vi "threshold-icator -scany.vi"(6 "first time":bool=TRUE, 7 "requested size":i32=1, 10 "gamma":dbl, 11 "omega":dbl) -> (0 "last peak":dbl, 1 "new peak":bool, 2 "gamma array":dbl[](array[numeric]), 3 "omega array":dbl[](array[numeric]))   [LabVIEW 2010]
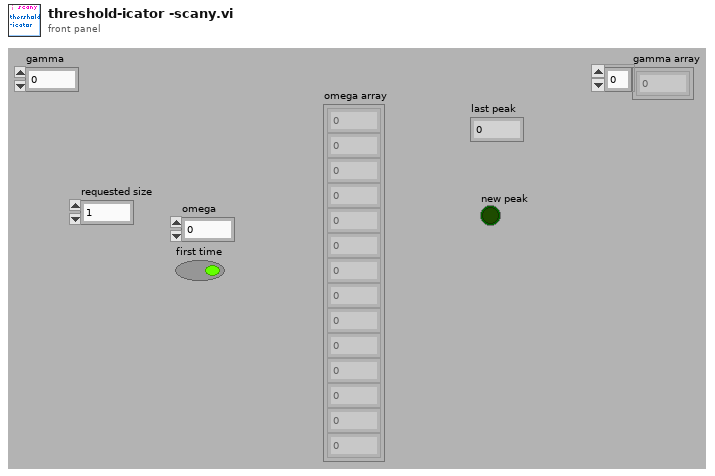
[diagram p1: front panel]
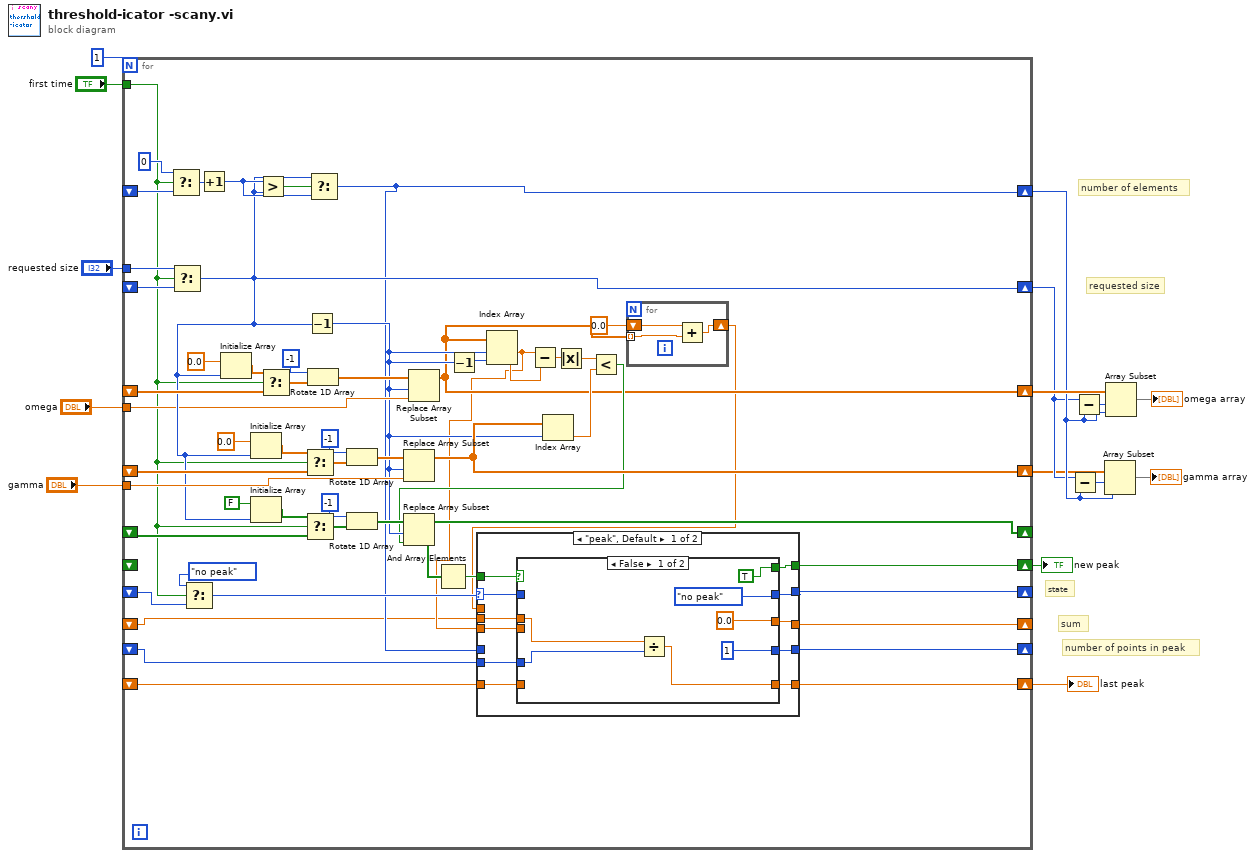
[diagram p0: block diagram]
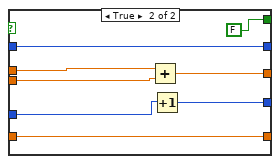
[diagram p2: hidden frame]
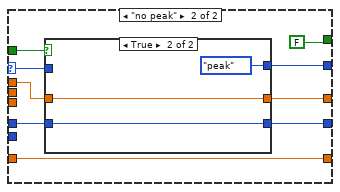
[diagram p3: hidden frame]
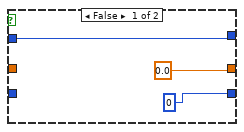
[diagram p4: hidden frame]
diagram:
  # "number of points in peak"
  # "sum"
  # "state"
  # "requested size"
  # "number of elements"
  n1 = for {
    N: 1 -> [_]
    tunnel: "first time" -> [w30]
    shift-right: [w22] -> w6
    shift-left: _ -> [w69]
    tunnel: "requested size" -> [w60]
    tunnel: "omega" -> [w37]
    shift-right: [w25] -> w11
    shift-left: _ -> [w65]
    shift-right: [w42] -> w5
    shift-left: _ -> [w59]
    shift-right: [w32] -> _
    shift-left: _ -> [w50]
    shift-right: [w36] -> w4
    shift-left: _ -> [w52]
    tunnel: "gamma" -> [w49]
    shift-right: [w28] -> _
    shift-left: _ -> [w41]
    shift-right: [w17] -> w1
    shift-left: _ -> [w16]
    shift-right: [w31] -> w2
    shift-left: _ -> [_]
    shift-right: [w23] -> _
    shift-left: _ -> [w19]
    shift-right: [w21] -> _
    shift-left: _ -> [w18]
    n2 = Select(t=0, s=w30, f=w69) -> (s? t:f=w67:i32)
    n3 = Select(t=w60, s=w30, f=w59) -> (s? t:f=w42:i32)
    n4 = Select(t=enum16{"peak", "no peak"}."no peak" ("Enum"), s=w30, f=w50) -> (s? t:f=w48:enum16{"peak", "no peak"})
    n5 = Increment(x=w67) -> (x+1=w66:i32)
    n6 = Initialize Array(0.0, w42) -> (w61:dbl[])
    n7 = Initialize Array(0.0, w42) -> (w56:dbl[])
    n8 = Initialize Array(FALSE, w42) -> (w47:bool[])
    n9 = Greater?(x=w66, y=w42) -> (0:w68:bool)
    n10 = Select(t=w61, s=w30, f=w65) -> (s? t:f=w58:dbl[])
    n11 = Select(t=w56, s=w30, f=w52) -> (s? t:f=w55:dbl[])
    n12 = Select(t=w47, s=w30, f=w41) -> (s? t:f=w46:bool[])
    n13 = Decrement(x=w42) -> (x-1=w35:i32)
    n14 = Rotate 1D Array(1:w58, 2:-1 ("n")) -> (0:w63:dbl[])
    n15 = Select(t=w42, s=w68, f=w66) -> (s? t:f=w22:i32)
    n16 = Rotate 1D Array(1:w55, 2:-1 ("n")) -> (0:w53:dbl[])
    n17 = Rotate 1D Array(1:w46, 2:-1 ("n")) -> (0:w44:bool[])
    n18 = Replace Array Subset(array=w53, new element=w49, index=w35) -> (w36:dbl[])
    n19 = Replace Array Subset(array=w63, new element=w37, index=w35) -> (w25:dbl[])
    n20 = Decrement(x=w35) -> (x-1=w40:i32)
    n21 = Index Array(array=w25, index #1=w35, index #2=w40) -> (element #1=w20:dbl, element #2=w29:dbl)
    n22 = Subtract(x=w20, y=w29) -> (x-y=w39:dbl)
    n23 = Index Array(array=w36, index=w35) -> (element=w34:dbl)
    n24 = Absolute Value(x=w39) -> (abs(x)=w38:dbl)
    n25 = Less?(x=w38, y=w34) -> (x < y?=w33:bool)
    n26 = Replace Array Subset(array=w44, new element=w33, index=w35) -> (w28:bool[])
    n27 = And Array Elements(Boolean array=w28) -> (logical AND=w27:bool)
    n28 = for {
      tunnel: w25 -> [w72] mode=indexing
      shift-right: [w71] -> w24
      shift-left: 0.0 -> [w73]
      n29 = Add(x=w73, y=w72) -> (x+y=w71:dbl)
    }
    n30 = case shown="\"peak\", Default" w48 {
      selector: w48 -> [w83 w107]
      tunnel: [w84 w108] -> w32
      tunnel: [w82 FALSE] -> w31
      tunnel: w27 -> [w81 w105]
      tunnel: w24 -> [_ w104]
      tunnel: [w78 w103] -> w23
      tunnel: w22 -> [_ w102]
      tunnel: [w76 w101] -> w21
      tunnel: w20 -> [w80 _]
      tunnel: w19 -> [w79 _]
      tunnel: w18 -> [w77 _]
      tunnel: [w75 w100] -> w17
      tunnel: w16 -> [w74 w100]
      frame "peak", Default {
        n31 = case shown="False" w81 {
          tunnel: [enum16{"peak", "no peak"}."no peak" ("Enum") w99] -> w84
          tunnel: w83 -> [_ w99]
          tunnel: [TRUE FALSE] -> w82
          tunnel: w80 -> [_ w97]
          tunnel: w79 -> [w89 w96]
          tunnel: [0.0 w95] -> w78
          tunnel: w77 -> [w88 w94]
          tunnel: [1 w93] -> w76
          tunnel: [w87 w92] -> w75
          tunnel: w74 -> [_ w92]
          frame False {
            n32 = Divide(x=w89, y=w88) -> (x/y=w87:dbl)
          }
          frame True {
            n33 = Add(x=w96, y=w97) -> (x+y=w95:dbl)
            n34 = Increment(x=w94) -> (x+1=w93:i32)
          }
        }
      }
      frame "no peak" {
        n35 = case shown="True" w105 {
          tunnel: [w111 enum16{"peak", "no peak"}."peak" ("Enum")] -> w108
          tunnel: w107 -> [w111 _]
          tunnel: w104 -> [_ w113]
          tunnel: [0.0 w113] -> w103
          tunnel: w102 -> [_ w112]
          tunnel: [0 w112] -> w101
          frame False {
          }
          frame True {
          }
        }
      }
    }
  }
  "last peak" <- w1
  "new peak" <- w2
  n36 = Subtract(x=w5, y=w6) -> (x-y=w8:i32)
  n37 = Subtract(x=w5, y=w6) -> (x-y=w9:i32)
  n38 = Array Subset(array=w4, index=w8, length=w6) -> (→"gamma array":dbl[])
  n39 = Array Subset(array=w11, index=w9, length=w6) -> (→"omega array":dbl[])
